vi "Global 5.vi"() -> ()   [LabVIEW 2015]
panel:
  in  "i":dbl
  in  "Saved_Hour":dbl
  in  "IsEclipse":bool
  out "Channel2_OFF":bool
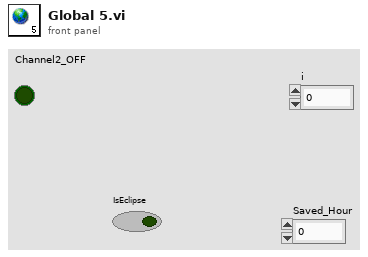
[diagram p1: front panel]
diagram:
